vi "SavePostPreList.vi"(8 "error in (no error)":errorcluster, 9 "Data":i32[][][](array[numeric]), 10 "Name File":string, 11 "Store Path":path) -> (0 "error out":errorcluster)   [LabVIEW 2013]
uses:
  <vilib>/Utility/xml.llb/Write to XML File(string).vi
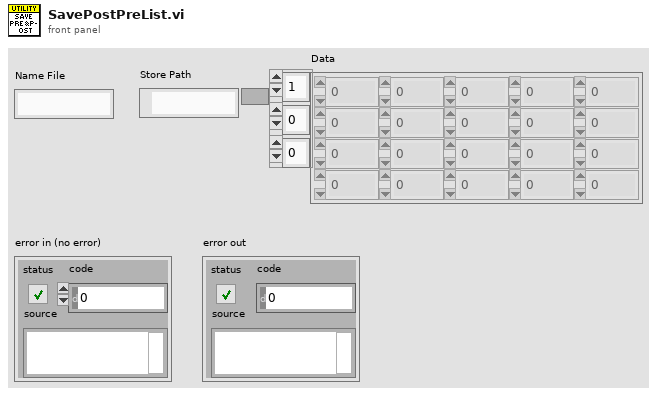
[diagram p1: front panel]
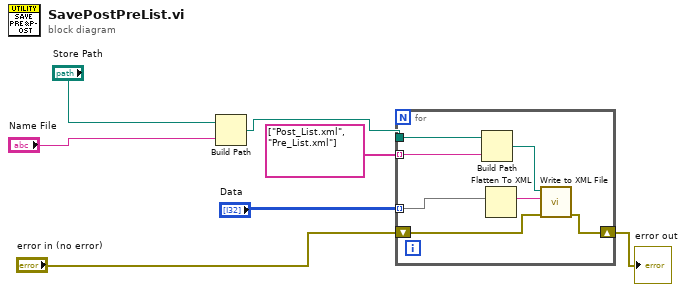
[diagram p0: block diagram]
diagram:
  n1 = Build Path(base path="Store Path", name or relative path="Name File") -> (appended path=w5:path)
  n2 = for {
    tunnel: "Data" -> [w14] mode=indexing
    tunnel: string[] ["Post_List.xml", "Pre_List.xml"] -> [w13] mode=indexing
    tunnel: w5 -> [w12]
    shift-right: [w8] -> w6
    shift-left: "error in (no error)" -> [w9]
    n3 = Build Path(base path=w12, name or relative path=w13) -> (appended path=w11:path)
    n4 = Flatten To XML(anything=w14) -> (xml string=w10:string)
    n5 = call-poly <vilib>:"Write to XML File.vi"("error in (no error)"=w9, "XML Input"=w10, "XML File Path"=w11) -> ("error out"=w8:errorcluster)  [unwired: 6 in, 2 out]
  }
  "error out" <- w6
